vi "FGV_Data.vi"(7 "Action_Data":T1, 8 "error in":errorcluster, 10 "Data In":cluster{"Data name":string, "Data":variant}, 11 "Data name":string) -> (0 "error out":errorcluster, 1 "Data Array out":cluster{"Data name":string, "Data":variant}[](array[cluster]), 2 "Data  Out":cluster{"Data name":string, "Data":variant})   [LabVIEW 2015]
uses:
  <userlib>/FGV/control/Control_Data.ctl
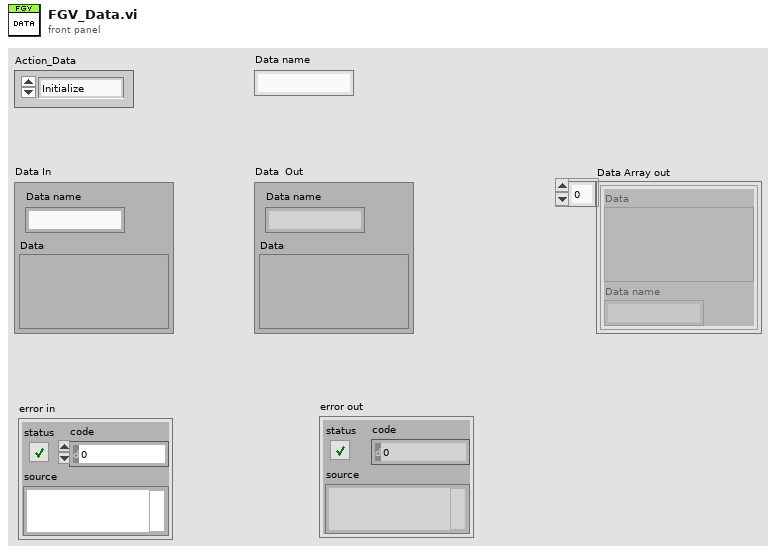
[diagram p1: front panel]
types:
  T1 = typedef "Control_Data.ctl" = enum16{"Initialize", "Get Data", "Set Data", "Delete Data", "Idle"}
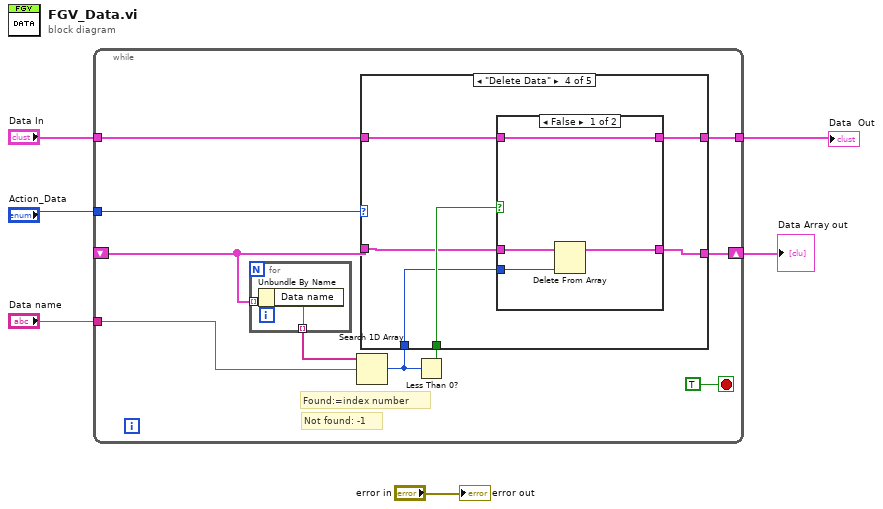
[diagram p0: block diagram]
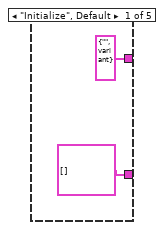
[diagram p2: hidden frame]
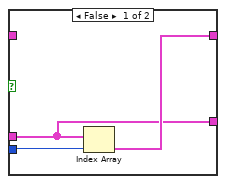
[diagram p4: hidden frame]
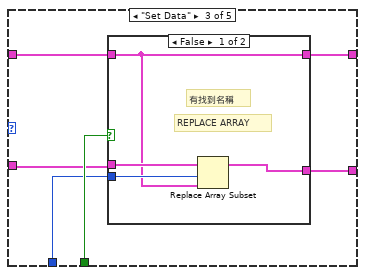
[diagram p5: hidden frame]
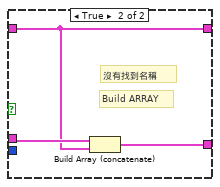
[diagram p6: hidden frame]
diagram:
  n1 = while {
    tunnel: "Action_Data" -> [w16]
    tunnel: "Data In" -> [w14]
    tunnel: [w13] -> w3
    shift-right: [w12] -> w2
    shift-left: _ -> [w11]
    tunnel: "Data name" -> [w9]
    stop <- TRUE stop-if-true
    # "Not found: -1"
    # "Found:=index number"
    n2 = for {
      tunnel: w11 -> [w18] mode=indexing
      tunnel: [w17] -> w10 mode=indexing
      n3 = Unbundle By Name(w18) -> ("Data name"=w17:string)
    }
    n4 = Search 1D Array(1D array=w10, element=w9) -> (index of element=w7:i32)  [unwired: 1 in]
    n5 = Less Than 0?(x=w7) -> (x < 0?=w8:bool)
    n6 = case shown="\"Delete Data\"" w16 {
      tunnel: w14 -> [_ w21 w32 w45 w58]
      tunnel: [cluster{"Data name":string, "Data":variant} {"Data name"="", "Data"=variant} ("Data In") w23 w33 w46 w58] -> w13
      tunnel: [cluster{"Data name":string, "Data":variant}[] [] w22 w34 w47 w57] -> w12
      tunnel: w11 -> [_ w25 w35 w49 w57]
      tunnel: w8 -> [_ w26 w37 w50 _]
      tunnel: w7 -> [_ w24 w36 w48 _]
      frame "Initialize", Default {
      }
      frame "Get Data" {
        n7 = case shown="True" w26 {
          tunnel: w25 -> [w27 w31]
          tunnel: w24 -> [w29 _]
          tunnel: [w28 w30] -> w23
          tunnel: [w27 w31] -> w22
          tunnel: w21 -> [_ w30]
          frame False {
            n8 = Index Array(array=w27, index=w29) -> (element=w28:cluster{"Data name":string, "Data":variant})
          }
          frame True {
          }
        }
      }
      frame "Set Data" {
        n9 = case shown="False" w37 {
          tunnel: w36 -> [w41 _]
          tunnel: w35 -> [w40 w44]
          tunnel: [w39 w43] -> w34
          tunnel: [w38 w42] -> w33
          tunnel: w32 -> [w38 w42]
          frame False {
            # "REPLACE ARRAY"
            # "有找到名稱"
            n10 = Replace Array Subset(array=w40, new element=w38, index=w41) -> (w39:cluster{"Data name":string, "Data":variant}[])
          }
          frame True {
            # "Build ARRAY"
            # "沒有找到名稱"
            n11 = Build Array (concatenate)(w44, w42) -> (w43:cluster{"Data name":string, "Data":variant}[])
          }
        }
      }
      frame "Delete Data" {
        n12 = case shown="False" w50 {
          tunnel: w49 -> [w54 w56]
          tunnel: w48 -> [w51 _]
          tunnel: [w53 w56] -> w47
          tunnel: [w52 w55] -> w46
          tunnel: w45 -> [w52 w55]
          frame False {
            n13 = Delete From Array(array=w54, index=w51) -> (array with subset deleted=w53:cluster{"Data name":string, "Data":variant}[])  [unwired: 1 in, 1 out]
          }
          frame True {
          }
        }
      }
      frame "Idle" {
      }
    }
  }
  "Data  Out" <- w3
  "Data Array out" <- w2
  "error out" <- "error in"
